vi "SwerveDriveSetWheelAuto.vi"(8 "error in (no error)":errorcluster, 9 "Swerve Drive Module States":T3 {"Angle"."SIN" format="%13.4f"; "Angle"."COS" format="%13.4f"; "Angle"."VALUE" format="%13.4f"}, 10 "Swerve Demand":T1[](array[typedef]) {"Angle"."SIN" format="%13.4f"; "Angle"."COS" format="%13.4f"; "Angle"."VALUE" format="%13.4f"}, 11 "SwerveDriveDevRef 2":T4={"DevStatus"={"status"=FALSE, "code"=0, "source"=""}, "TurnMotors[]"=[], "Square Inputs"=FALSE, "Max Output"=1.0, "DriveMotors[]"=[], "WheelOffset[]"=[], "SwerveSensors[]"=[], "RobotSize"={"Width"=[], "Length"=[], "Center"=[]}}) -> (0 "error out":errorcluster, 2 "Swerve Drive Module States Out":T3 {"Angle"."SIN" format="%13.4f"; "Angle"."COS" format="%13.4f"; "Angle"."VALUE" format="%13.4f"}, 3 "SwerveDriveDevRef":T4={"DevStatus"={"status"=FALSE, "code"=0, "source"=""}, "TurnMotors[]"=[], "Square Inputs"=FALSE, "Max Output"=1.0, "DriveMotors[]"=[], "WheelOffset[]"=[], "SwerveSensors[]"=[], "RobotSize"={"Width"=[], "Length"=[], "Center"=[]}})   [LabVIEW 2019]
uses:
  Swerve Drive.lvlib
  <vilib>/Rock Robotics/WPI/ThirdParty/REV Robotics/SPARK MAX/Typedef/Spark MAX Control Type.ctl
  <vilib>/Rock Robotics/SystemInterfaces/DIO/FPGA_DIOPWMChannel.ctl
  <vilib>/Rock Robotics/WPI/PWM/WPI_PWMDeadband.ctl
  <vilib>/Rock Robotics/WPI/MotorControl/WPI_MotorControlType.ctl
  <vilib>/Rock Robotics/SystemInterfaces/DIO/FPGA_DIOChannel.ctl
  <vilib>/Rock Robotics/WPI/MotorControl/WPI_MotorControlDeviceRef.ctl
  <vilib>/Rock Robotics/SystemInterfaces/AI/FPGA_AIChannel.ctl
  SwerveDriveDevRef.ctl
  <vilib>/Rock Robotics/WPI/ThirdParty/JAS_Junk/TrajLib/ROTATION2D.ctl
  <vilib>/Rock Robotics/WPI/ThirdParty/JAS_Junk/TrajLib/Trajectory_Library.lvlib
  <vilib>/Rock Robotics/WPI/ThirdParty/JAS_Junk/TrajLib/SWERVE_DRIVE_MODULE_STATE.ctl
  SwerveDriveModuleStates.ctl
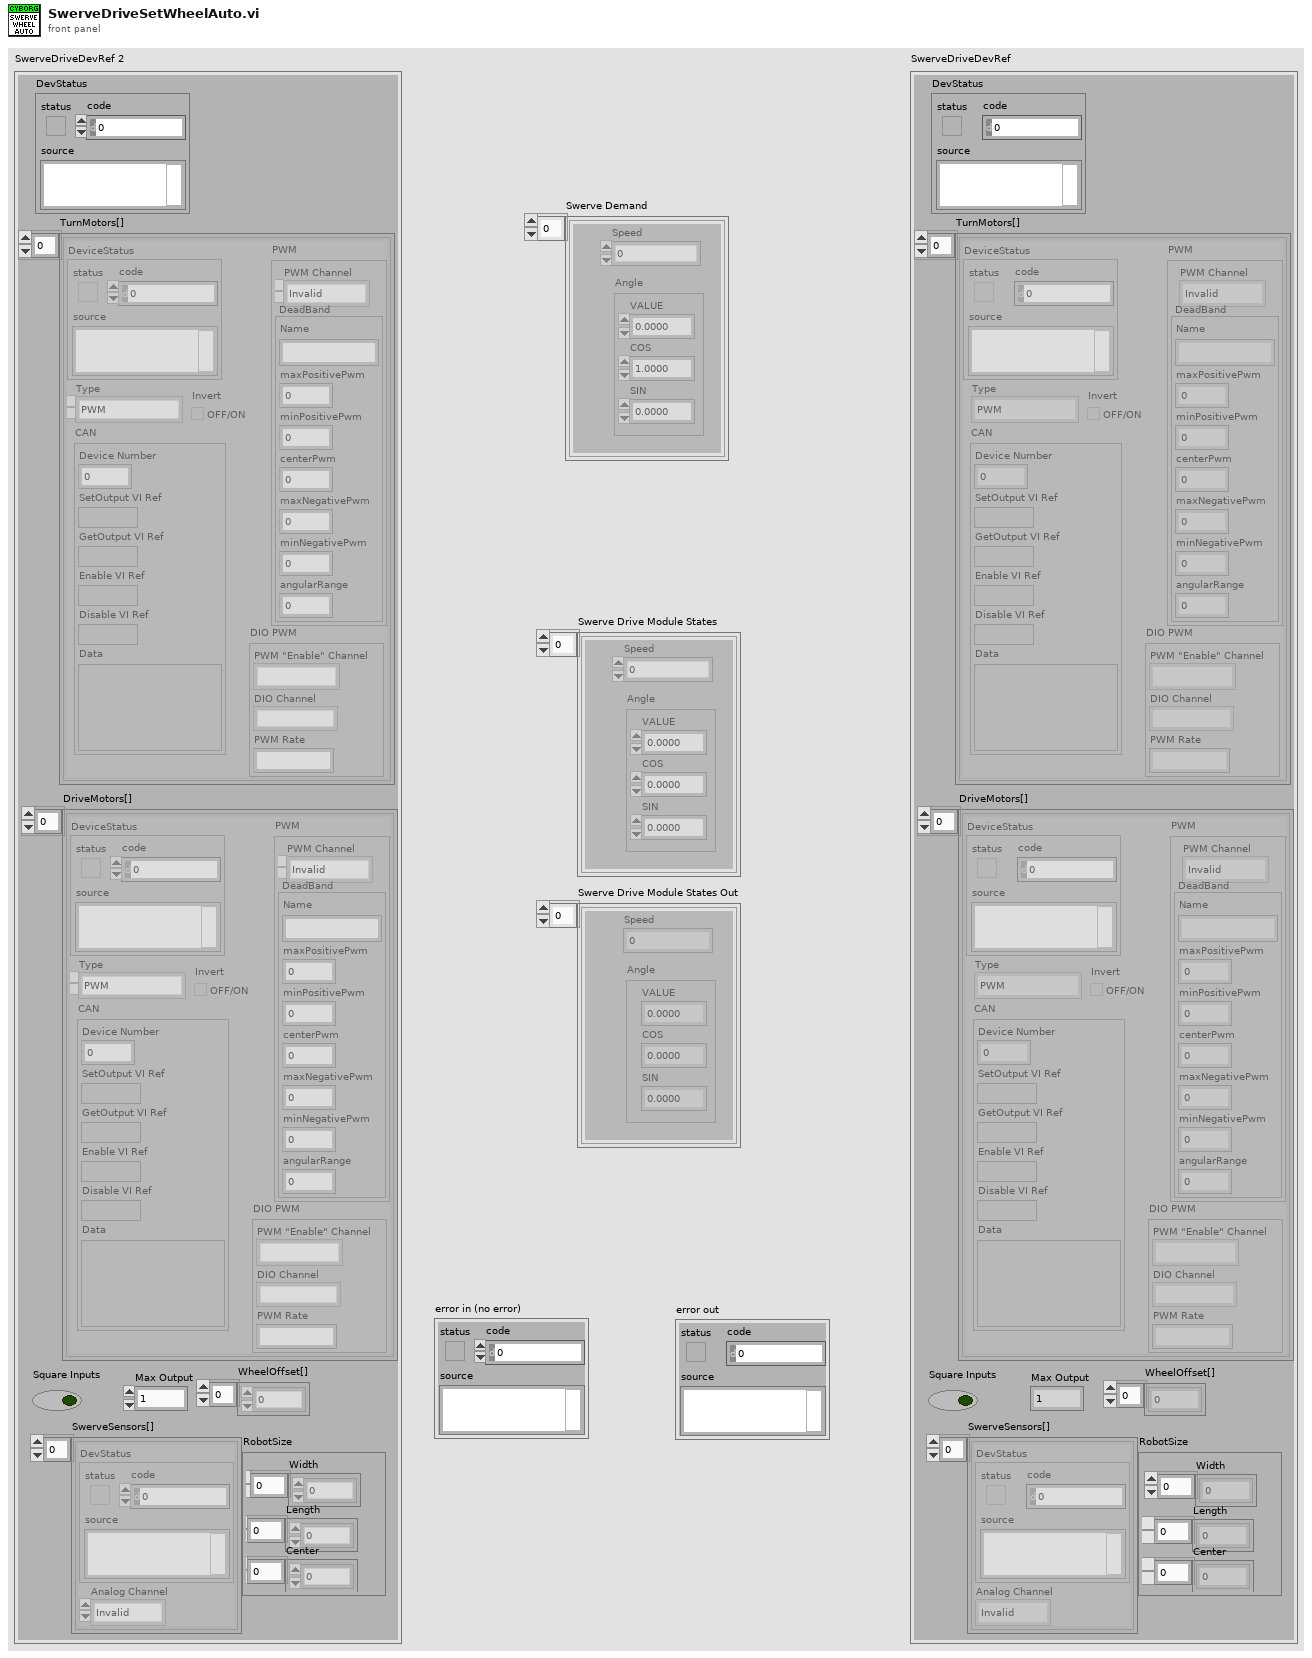
[diagram p1: front panel]
types:
  T1 = typedef "Trajectory_Library.lvlib/SWERVE_DRIVE_MODULE_STATE.ctl" = cluster{"Speed":dbl, "Angle":T2}
  T2 = typedef "Trajectory_Library.lvlib/ROTATION2D.ctl" = cluster{"VALUE":dbl, "COS":dbl, "SIN":dbl}
  T3 = typedef "SwerveDriveModuleStates.ctl" = T1[]
  T4 = typedef "Swerve Drive.lvlib/SwerveDriveDevRef.ctl" = cluster{"DevStatus":errorcluster, "TurnMotors[]":T5[], "Square Inputs":bool, "Max Output":dbl, "DriveMotors[]":T5[], "WheelOffset[]":dbl[], "SwerveSensors[]":cluster{"DevStatus":errorcluster, "Analog Channel":T10}[], "RobotSize":cluster{"Width":dbl[], "Length":dbl[], "Center":dbl[]}}
  T5 = typedef "WPI_MotorControlDeviceRef.ctl" = cluster{"DeviceStatus":errorcluster, "Type":T6, "PWM":cluster{"PWM Channel":T7, "DeadBand":T8}, "CAN":cluster{"Device Number":u8, "SetOutput VI Ref":variant, "GetOutput VI Ref":variant, "Enable VI Ref":variant, "Disable VI Ref":variant, "Data":variant}, "Invert":bool, "DIO PWM":cluster{"PWM \"Enable\" Channel":T7, "DIOChannel":T9, "PWM Rate":dbl}}
  T6 = typedef "WPI_MotorControlType.ctl" = enum16{"PWM", "CAN", "DIO PWM"}
  T7 = typedef "FPGA_DIOPWMChannel.ctl" = enum8{"PWM 0", "PWM 1", "PWM 2", "PWM 3", "PWM 4", "PWM 5", "PWM 6", "PWM 7", "PWM 8", "PWM 9", "PWM MXP 0", "PWM MXP 1", "PWM MXP 2", "PWM MXP 3", "PWM MXP 4", "PWM MXP 5", "PWM MXP 6", "PWM MXP 7", "PWM MXP 8", "PWM MXP 9", "Invalid"}
  T8 = typedef "WPI_PWMDeadband.ctl" = cluster{"Name":string, "maxPositivePwm":i32, "minPositivePwm":i32, "centerPwm":i32, "maxNegativePwm":i32, "minNegativePwm":i32, "angularRange":u16}
  T9 = typedef "FPGA_DIOChannel.ctl" = enum8{"DIO 0", "DIO 1", "DIO 2", "DIO 3", "DIO 4", "DIO 5", "DIO 6", "DIO 7", "DIO 8", "DIO 9", "DIO MXP 0", "DIO MXP 1", "DIO MXP 2", "DIO MXP 3", "DIO MXP 4", "DIO MXP 5", "DIO MXP 6", "DIO MXP 7", "DIO MXP 8", "DIO MXP 9", "DIO MXP 10", "DIO MXP 11", "DIO MXP 12", "DIO MXP 13", "DIO MXP 14", "DIO MXP 15", "SPI Port CS1", "SPI Port CS2", "SPI Port CS3", "SPI Port MISO", "SPI Port MOSI", "Invalid"}
  T10 = typedef "FPGA_AIChannel.ctl" = enum8{"AI 0", "AI 1", "AI 2", "AI 3", "AI MXP 0", "AI MXP 1", "AI MXP 2", "AI MXP 3", "Invalid"}
  T11 = typedef "Spark MAX Control Type.ctl" = enum16{"Percent VBus", "Voltage", "Velocity", "Position", "Smart Motion", "Current", "Smart Velocity"}
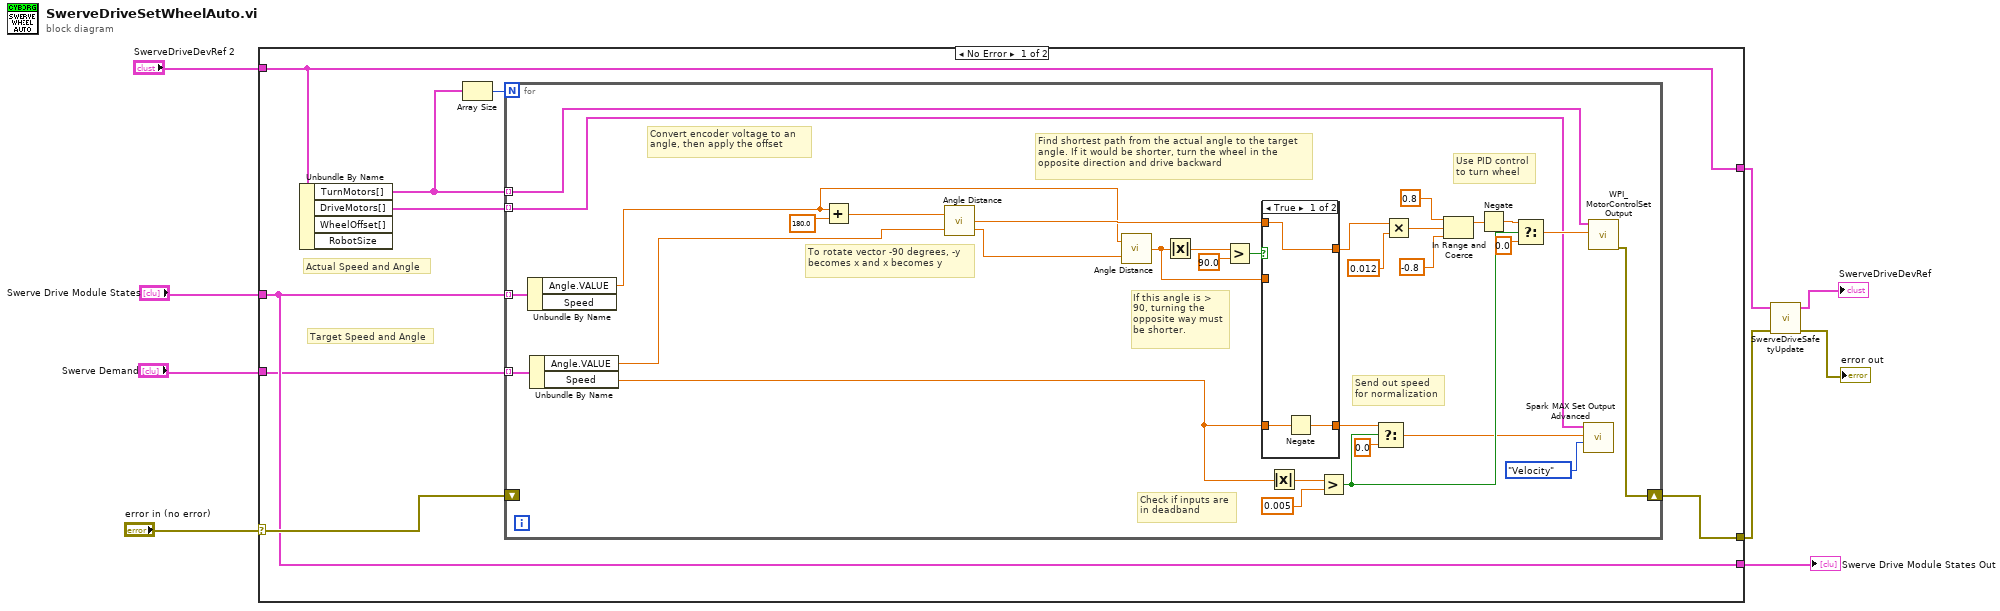
[diagram p0: block diagram]
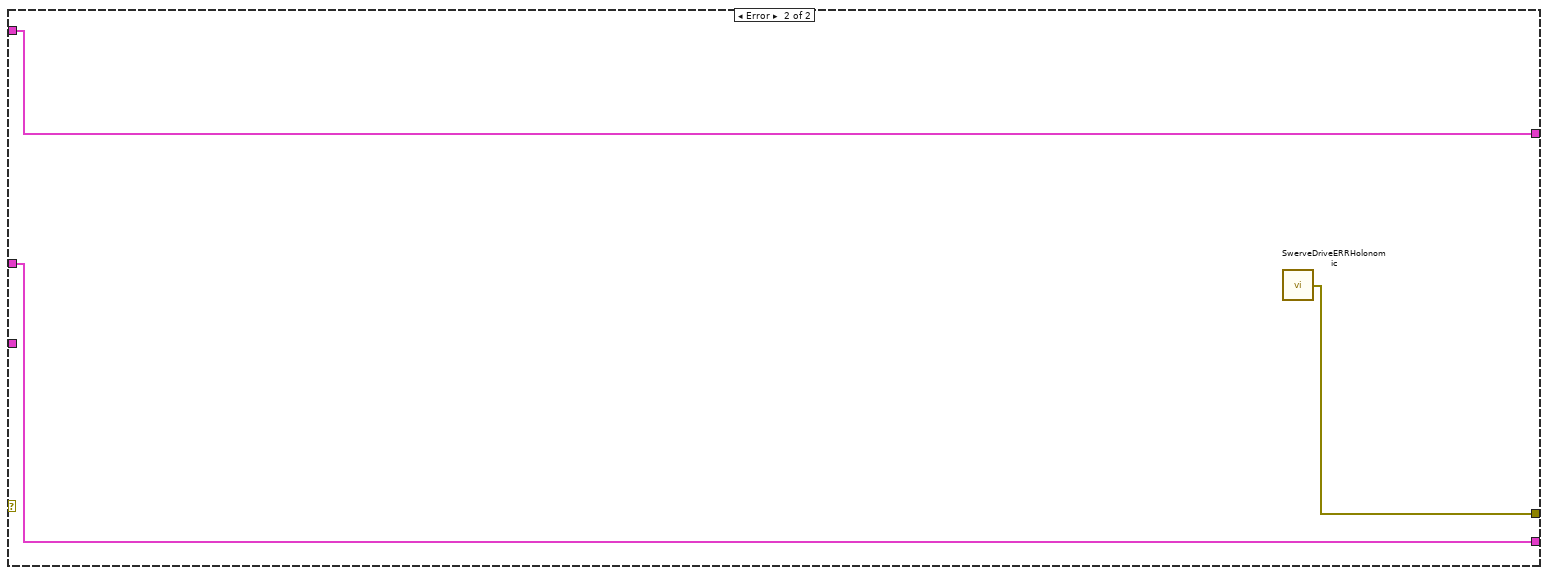
[diagram p3: hidden frame]
diagram:
  n1 = case shown="No Error" "error in (no error)" {
    selector: "error in (no error)" -> [w17 _]
    tunnel: "SwerveDriveDevRef 2" -> [w15 w56]
    tunnel: [w15 w56] -> w7
    tunnel: [w16 w55] -> w5
    tunnel: "Swerve Demand" -> [w10 _]
    tunnel: "Swerve Drive Module States" -> [w11 w54]
    tunnel: [w11 w54] -> w2
    frame No Error {
      # "Actual Speed and Angle"
      # "Target Speed and Angle"
      n2 = Unbundle By Name(w15) -> ("TurnMotors[]"=w12:T5[], "DriveMotors[]"=w14:T5[])  [unwired: 2 out]
      n3 = Array Size(array=w12) -> (size(s)=w13:i32)
      n4 = for {
        N: w13 -> [_]
        shift-right: [w34] -> w16
        shift-left: w17 -> [_]
        tunnel: w12 -> [w35] mode=indexing
        tunnel: w14 -> [w24] mode=indexing
        tunnel: w11 -> [w19] mode=indexing
        tunnel: w10 -> [w18] mode=indexing
        # "To rotate vector -90 degrees, -y becomes x and x becomes y"
        # "Send out speed\nfor normalization"
        # "Check if inputs are\nin deadband"
        # "Convert encoder voltage to an angle, then apply the offset"
        # "If this angle is > 90, turning the opposite way must be shorter."
        # "Use PID control\nto turn wheel"
        # "Find shortest path from the actual angle to the target angle. If it would be shorter, turn the wheel in the opposite direction and drive backward"
        n5 = Unbundle By Name(w19) -> ("Angle.VALUE"=w22:dbl)  [unwired: 1 out]
        n6 = Unbundle By Name(w18) -> ("Angle.VALUE"=w21:dbl, "Speed"=w20:dbl)
        n7 = Add(x=w22, y=180.0 ("f")) -> (x+y=w43:dbl)
        n8 = call "Angle Distance.vi"("target angle"=w21, "current angle"=w43) -> ("distance"=w36:dbl)
        n9 = call "Angle Distance.vi"("target angle"=w21, "current angle"=w22) -> ("distance"=w46:dbl)
        n10 = Absolute Value(x=w46) -> (abs(x)=w47:dbl)
        n11 = Greater?(x=w47, y=90.0) -> (0:w40:bool)
        n12 = case shown="True" w40 {
          tunnel: w36 -> [w49 _]
          tunnel: w46 -> [_ w53]
          tunnel: [w50 w52] -> w42
          tunnel: w20 -> [w51 w52]
          tunnel: [w49 w53] -> w29
          frame True {
            n13 = Negate(x=w51) -> (-x=w50:dbl)
          }
          frame False {
          }
        }
        n14 = Absolute Value(x=w20) -> (abs(x)=w27:dbl)
        n15 = Greater?(x=w27, y=0.005) -> (0:w39:bool)
        n16 = Select(t=w42, s=w39, f=0.0) -> (s? t:f=w25:dbl)
        n17 = Multiply(x=w29, y=0.012) -> (x*y=w32:dbl)
        n18 = In Range and Coerce(upper limit=0.8, x=w32, lower limit=-0.8) -> (coerced(x)=w33:dbl)  [unwired: 1 out]
        n19 = Negate(x=w33) -> (-x=w38:dbl)
        n20 = Select(t=w38, s=w39, f=0.0) -> (s? t:f=w45:dbl)
        n21 = call <vilib>:"Spark MAX Set Output Advanced.vi"("Control Mode"=Spark_MAX_Control_Type."Velocity", "Setpoint"=w25, "MotorControlDevRef"=w24) -> ()  [unwired: 7 in, 2 out]
        n22 = call <vilib>:"WPI_MotorControlSetOutput.vi"("Output"=w45, "MotorControlDevRef"=w35) -> ("error out"=w34:errorcluster)  [unwired: 7 in, 2 out]
      }
    }
    frame Error {
      n23 = call "SwerveDriveERRHolonomic.vi"() -> ("error out"=w55:errorcluster)
    }
  }
  "Swerve Drive Module States Out" <- w2
  n24 = call "SwerveDriveSafetyUpdate.vi"("error in (no error)"=w5, "SwerveDriveDevRef 2"=w7) -> ("error out"=→"error out":errorcluster, "SwerveDriveDevRef"=→"SwerveDriveDevRef":T4)  [unwired: 8 in]
